vi "Data from Channel 0 and Channel 1.vi"() -> (3 "Channels Data":i16[](array[numeric]))   [LabVIEW 2012]
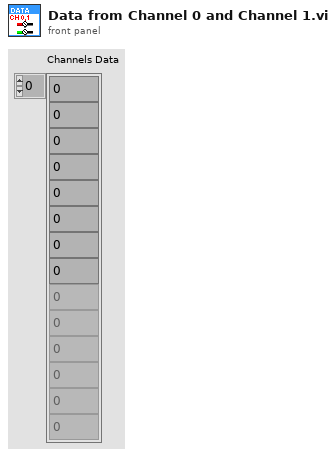
[diagram p1: front panel]
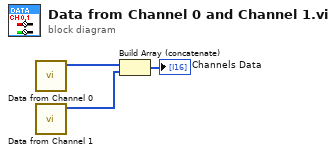
[diagram p0: block diagram]
diagram:
  n1 = call <userlib>:"Data from Channel 0.vi"() -> ("Channel Data"=w2:i16[])  [unwired: 11 in]
  n2 = call <userlib>:"Data from Channel 1.vi"() -> ("Channels Data"=w1:i16[])  [unwired: 11 in]
  n3 = Build Array (concatenate)(w2, w1) -> (→"Channels Data":i16[])
